vi "PH_SSAC.constructor.vi"(0 "name":string, 2 "data in":string, 5 "error in(no error)":errorcluster) -> (14 "i ref out":refnum<vi>, 16 "data out":string, 19 "error out":errorcluster)   [LabVIEW 2014, in "PH_SSAC.lvlib"]
doc: "This is the constructor of a class.\n\nLicense Agreement for this software:\n\nCopyright (C)\nGesellschaft für Schwerionenforschung, GSI\nPlanckstr. 1\n64291 Darmstadt\nGermany\n\nContact: D.Beck@gsi.de \n\nThis program is free software; you can redistribute it and/or modify it under the terms of the \nGNU General Public License as published by the Free Software Foundation; either version 2 of \nthe license, or (at your option) any later version.\n\nThis program is distributed in the hope that it will be useful, but WITHOUT ANY WARRANTY; \nwithout even the implied warranty of MERCHANTABILITY or FITNESS FOR A PARTICULAR PURPOSE. See the GNU General License for more details (http://www.gnu.org).\n\nGesellschaft für Schwerionenforschung, GSI\nPlanckstr. 1, 64291 Darmstadt, Germany\nFor all questions and ideas contact: M.Richter@gsi.de, H.Brand@gsi.de or D.Beck@gsi.de.\nLast update: 16-JUN-2004"
uses:
  PH_SSAC.lvlib
  CS_Core/CSSystem/CSSystemLib/CSSystemLib.lvlib
  CS_Core/CSObj/CSObj.lvlib
  PH_Basics/PH_PSDBWriter/PH_PSDBWriter.lvlib
  PH_Basics/PH_Img_BaseClass/PH_Img_BaseClass.lvlib
  PH_Basics/PH_Class/PH_Class.lvlib
  PH_Basics/PH_Common/PH_Common.lvlib
  PH_Basics/PH_StatusHandler/PH_StatusHandler.lvlib
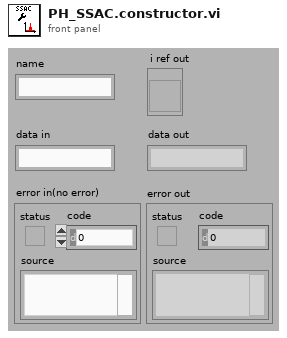
[diagram p1: front panel]
types:
  T1 = enum16{"SetAttribute", "GetAttribute", "CreateAttribute", "DestroyAttribute", "DestroyAllAtributes"}
  T2 = typedef "PH_SSAC.lvlib/PH_SSAC.i attribute.ctl" = cluster{"GUI Refs":cluster{"Delete":refnum<vi>, "Global On":refnum<vi>, "Cam Source":refnum<vi>, "Frame Main Signal":refnum<vi>, "Frame Background":refnum<vi>, "dt (Gauss smooth)":refnum<vi>, "Calibration Factor":refnum<vi>, "Background acquire":refnum<vi>, "Threshold":refnum<vi>, "Time evolution of mean pulse duration":refnum<vi>, "Mean Pulse Duration":refnum<vi>, "Main signal":refnum<vi>, "Current Pulse Duration":refnum<vi>, "Processed":refnum<vi>, "Saturation":refnum<vi>, "# for Average":refnum<vi>, "Position":refnum<vi>, "BG Status":refnum<vi>, "Save BG data":refnum<vi>, "Read BG Data":refnum<vi>, "Background Calibration Data":refnum<vi>}, "Images":cluster{"OP Image":T3, "GUI Image":T3, "PSDB Image":T3}, "Global On?":bool, "Frame Main":cluster{"x":u32, "dx":u32, "y":u32, "dy":u32}, "Frame Background":cluster{"x":u32, "dx":u32, "y":u32, "dy":u32}, "dt [fs]":dbl, "Calibration Factor [fs/pixel]":dbl, "Threshold":dbl, "Time evolution of mean pulse duration [fs]":dbl[], "Main Signal":cluster{"Time for Main":dbl[], "Signal":dbl[]}, "Processed":bool, "Current Pulse Duration [fs]":dbl, "# for Average":i32, "Position":i32, "Pulse Durations [fs]":dbl[], "BG":cluster{"Acquire?":bool, "Background Calibration Data":T4, "Save Data":bool}}
  T3 = typedef "IMAQ Image.ctl" = refnum<image>
  T4 = typedef "PH_SSAC.lvlib/PH_SSAC.Background Data.ctl" = cluster{"Date":string, "Time":string, "Frame Main":cluster{"x":u32, "dx":u32, "y":u32, "dy":u32}, "dt [fs]":dbl, "Calibration Factor [fs/pixel]":dbl, "Signal":dbl[], "Frame Background":cluster{"x":u32, "dx":u32, "y":u32, "dy":u32}}
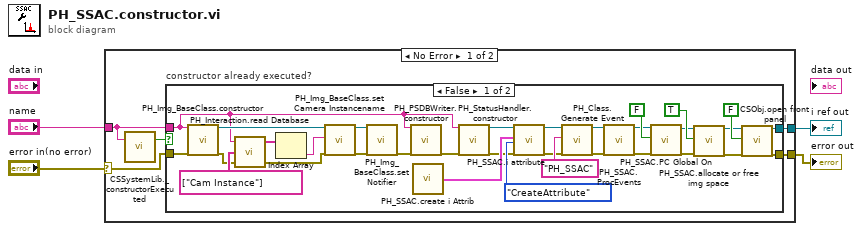
[diagram p0: block diagram]
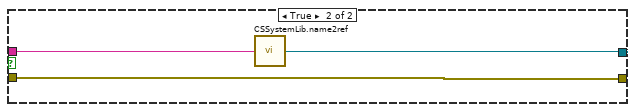
[diagram p2: hidden frame]
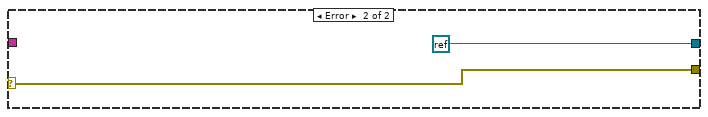
[diagram p3: hidden frame]
diagram:
  n1 = case shown="No Error" "error in(no error)" {
    selector: "error in(no error)" -> [w7 w45]
    tunnel: "name" -> [w6 _]
    tunnel: [w9 refnum<k0> refnum] -> w3
    tunnel: [w8 w45] -> w2
    frame No Error {
      n2 = call "CSSystemLib._constructorExecuted.vi"("name"=w6) -> ("constructor executed?"=w5:bool)  [unwired: 18 in]
      n3 = case "constructor already executed?" shown="False" w5 {
        tunnel: [w40 w43] -> w9
        tunnel: [w39 w42] -> w8
        tunnel: w7 -> [w41 w42]
        tunnel: w6 -> [w12 w44]
        frame False {
          n4 = call "PH_Img_BaseClass.constructor.vi"("name"=w12, "error in(no error)"=w41) -> ("i ref out"=w17:refnum<vi>, "error out"=w16:errorcluster)  [unwired: 15 in, 1 out]
          n5 = call "PH_Interaction.read Database.vi"("error in (no error)"=w16, "Strings to search for"=string[] ["Cam Instance"], "DB Entry to read"=w12) -> ("error out"=w15:errorcluster, "Values"=w19:string[])  [unwired: 1 in]
          n6 = Index Array(array=w19) -> (element=w18:string)  [unwired: 1 in]
          n7 = call "PH_Img_BaseClass.set Camera Instancename.vi"("i ref in"=w17, "Camera Instancename"=w18, "error in (no error)"=w15) -> ("i ref out"=w34:refnum<vi>, "error out"=w35:errorcluster)  [unwired: 15 in]
          n8 = call "PH_Img_BaseClass.set Notifier.vi"("i ref in"=w34, "error in"=w35) -> ("error out"=w21:errorcluster)  [unwired: 16 in, 1 out]
          n9 = call "PH_PSDBWriter.constructor.vi"("name"=w12, "error in"=w21) -> ("error out"=w28:errorcluster)  [unwired: 15 in, 2 out]
          n10 = call "PH_SSAC.create i Attrib.vi"() -> ("i Attr"=w31:T2)  [unwired: 1 in]
          n11 = call "PH_StatusHandler.constructor.vi"("name"=w12, "error in(no error)"=w28) -> ("i ref out"=w13:refnum<vi>, "error out"=w14:errorcluster)  [unwired: 15 in, 1 out]
          n12 = call "PH_SSAC.i attribute.vi"("VI Refnum"=w13, "CLASS.i attribute"=w31, "Action"=T1."CreateAttribute", "error in (no error)"=w14) -> ("VI Refnum out"=w30:refnum<vi>, "error out"=w29:errorcluster)  [unwired: 13 in, 1 out]
          n13 = call "PH_Class.Generate Event.vi"("i ref in"=w30, "Class"="PH_SSAC", "error in (no error)"=w29) -> ("i ref out"=w27:refnum<vi>, "error out"=w26:errorcluster)  [unwired: 15 in]
          n14 = call "PH_SSAC.ProcEvents.vi"("i ref in"=w27, "error in"=w26) -> ("i ref out"=w25:refnum<vi>, "error out"=w24:errorcluster)  [unwired: 16 in]
          n15 = call "PH_SSAC.PC Global On.vi"("i ref in"=w25, "Global On?"=FALSE, "error in (no error)"=w24) -> ("i ref out"=w10:refnum<vi>, "error out"=w11:errorcluster)  [unwired: 15 in]
          n16 = call "PH_SSAC.allocate or free img space.vi"("i ref in"=w10, "Allocate?"=TRUE, "error in (no error)"=w11) -> ("i ref out"=w23:refnum<vi>, "error out"=w22:errorcluster)  [unwired: 15 in]
          n17 = call "CSObj.open front panel.vi"("i ref in"=w23, "frontPanelOpen"=FALSE ("front panel open"), "error in (no error)"=w22) -> ("i ref out"=w40:refnum<vi>, "error out"=w39:errorcluster)  [unwired: 15 in]
        }
        frame True {
          n18 = call "CSSystemLib.name2ref.vi"("name"=w44) -> ("obj refnum"=w43:refnum<vi>)
        }
      }
    }
    frame Error {
    }
  }
  "i ref out" <- w3
  "error out" <- w2
